vi "Get Poller.vi"(8 "error in (no error)":errorcluster, 11 "input in":refnum<class "input.lvclass">) -> (0 "error out":errorcluster, 2 "input_poller.lvclass":refnum<class "input_poller.lvclass">, 3 "input out":refnum<class "input.lvclass">)   [LabVIEW 2015, in "input.lvclass"]
uses:
  input.lvclass
  input_poller/input_poller.lvclass
  input.lvclass/input.ctl
  input_poller/input_poller_queue/input_poller_queue.lvclass
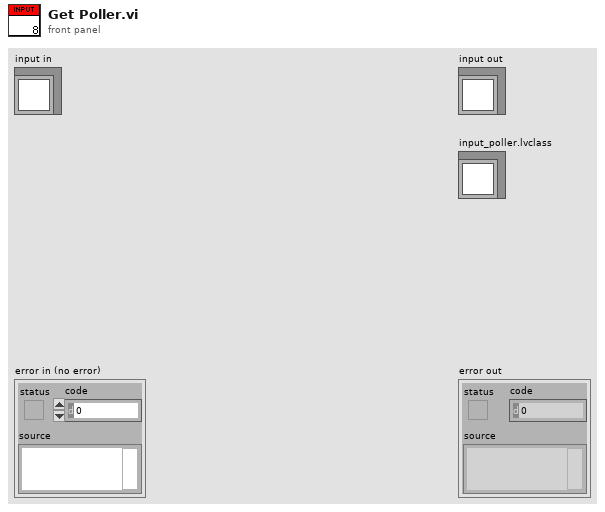
[diagram p1: front panel]
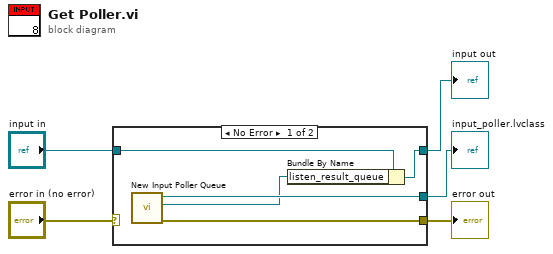
[diagram p0: block diagram]
diagram:
  n1 = case shown="No Error" "error in (no error)" {
    selector: "error in (no error)" -> [_ w12]
    tunnel: [w6 w12] -> w4
    tunnel: [w9 w11] -> w2
    tunnel: "input in" -> [w10 w11]
    tunnel: [w8 _] -> w1
    frame No Error {
      n2 = call "New Input Poller Queue.vi"() -> ("error out"=w6:errorcluster, "listen_result_queue"=w7:refnum<queue>, "input poller"=w8:refnum<class "input_poller_queue.lvclass">)  [unwired: 9 in]
      n3 = Bundle By Name(cluster=w10, "listen_result_queue"=w7) -> (w9:refnum<class "input.lvclass">)
    }
    frame Error {
    }
  }
  "error out" <- w4
  "input out" <- w2
  "input_poller.lvclass" <- w1
